vi "Running.vi"(7 "LabVIEW Web Service Request":refnum<class "Web Request.lvclass">) -> ()   [LabVIEW 2023]
uses:
  <vilib>/wsapi/Web Request.lvclass
  Bad Idea Globals.vi
panel:
  # "Use the Web Service Request input terminal to call the VIs on the Web Services palette. Do not remove it from the connector pane unless you don't need access to the palette."
  # "Each additional control wired to the connector pane will be available as an input in the URL. To include an indicator in terminal-mode output (the default setting), it must also be wired to the connector pane."
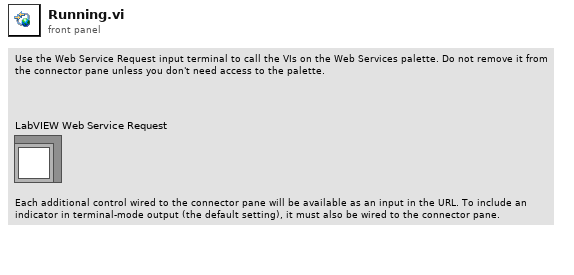
[diagram p1: front panel]
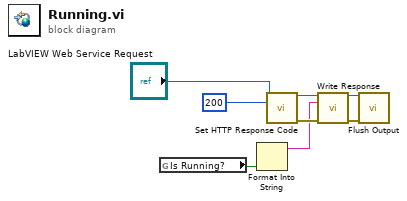
[diagram p0: block diagram]
diagram:
  n1 = global read "Bad Idea Globals.vi" "Is Running?"() -> (w2:bool)
  n2 = Format Into String(w2) -> (resulting string=w1:string)  [unwired: 3 in, 1 out]
  n3 = call <vilib>:"Set HTTP Response Code.vi"("LabVIEW Web Service Request"="LabVIEW Web Service Request", "response code (200)"=200) -> ("LabVIEW Web Service Request out"=w8:refnum<class "Web Request.lvclass">, "error out"=w7:errorcluster)  [unwired: 12 in]
  n4 = call <vilib>:"Write Response.vi"("LabVIEW Web Service Request"=w8, "response string"=w1, "error in (no error)"=w7) -> ("LabVIEW Web Service Request out"=w6:refnum<class "Web Request.lvclass">, "error out"=w5:errorcluster)  [unwired: 11 in]
  n5 = call <vilib>:"Flush Output.vi"("LabVIEW Web Service Request"=w6, "error in (no error)"=w5) -> ()  [unwired: 12 in, 2 out]
